vi "String to char Array.vi"(1 "Input":string) -> (0 "Array":string[](array[string]))   [LabVIEW 2020]
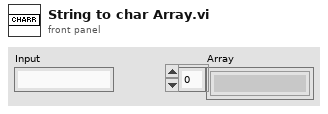
[diagram p1: front panel]
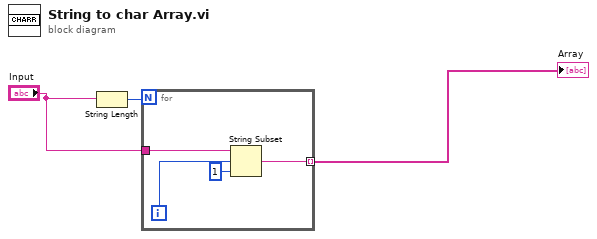
[diagram p0: block diagram]
diagram:
  n1 = String Length(string="Input") -> (length=w2:i32)
  n2 = for {
    N: w2 -> [_]
    tunnel: "Input" -> [w7]
    tunnel: [w4] -> w3 mode=indexing
    i -> [w5]
    n3 = String Subset(string=w7, offset (0)=w5, length (rest)=1 ("length (rest)")) -> (substring=w4:string)
  }
  "Array" <- w3
